vi "Median filter.vi"(11 "Rawdata":i32) -> (3 "Filtered element":i32)   [LabVIEW 2016]
doc: "Input\nRawdata\n\nOutput\nFiltered value\n\nThis VI implements a point to point median filter of rank 7. If one would like to change to the rank, you will need to set an odd number and change the size of the initial array for the feedback loop."
panel:
  in  "Middle":i32=4
  in  "Size of filter":i32=7
  # "Number of points to find median from,\nyou are best of choosing and odd number\nsince you want to avoid division on FPGA."
  # "Middle of size of filter"
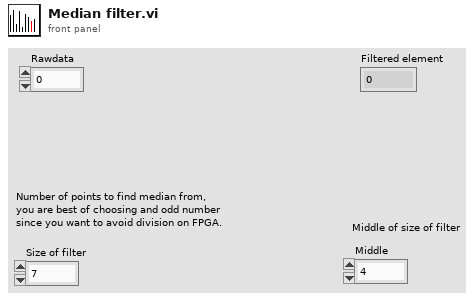
[diagram p1: front panel]
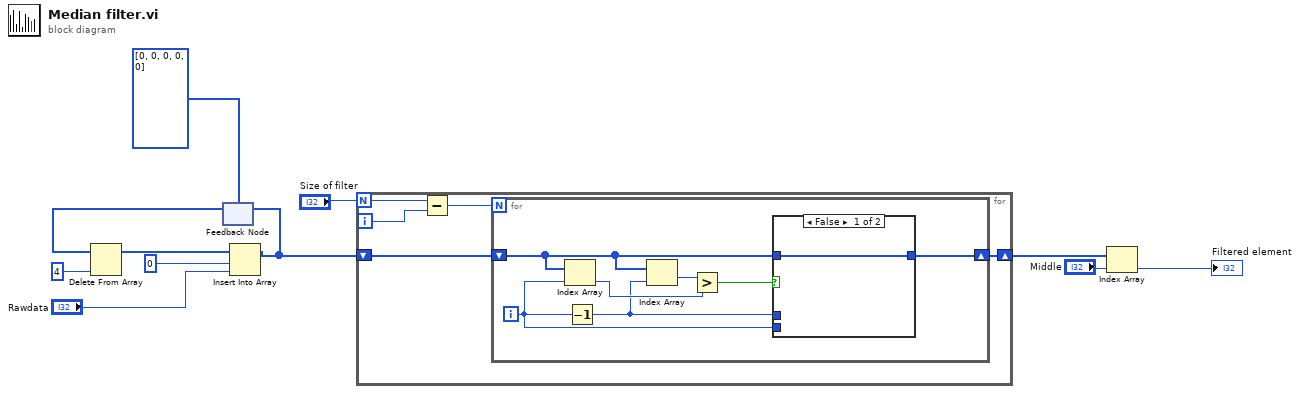
[diagram p0: block diagram]
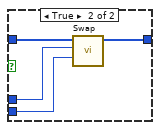
[diagram p2: hidden frame]
diagram:
  n1 = feedback #1(i32[] [0, 0, 0, 0, 0]) -> (w3:i32[])
  n2 = Delete From Array(array=w3, index=4) -> (array with subset deleted=w2:i32[])  [unwired: 1 in, 1 out]
  n3 = Insert Into Array(array=w2, index=0, new element="Rawdata") -> (w1:i32[])
  n4 = feedback-in #1(w1) -> ()
  n5 = for {
    N: "Size of filter" -> [w16]
    shift-right: [w12] -> w11
    shift-left: w1 -> [w13]
    i -> [w15]
    n6 = Subtract(x=w16, y=w15) -> (x-y=w14:i32)
    n7 = for {
      N: w14 -> [_]
      shift-right: [w19] -> w12
      shift-left: w13 -> [w23]
      i -> [w18]
      n8 = Index Array(array=w23, index=w18) -> (element=w21:i32)
      n9 = Decrement(x=w18) -> (x-1=w17:i32)
      n10 = Index Array(array=w23, index=w17) -> (element=w22:i32)
      n11 = Greater?(x=w22, y=w21) -> (0:w20:bool)
      n12 = case shown="False" w20 {
        tunnel: w23 -> [w24 w28]
        tunnel: w17 -> [_ w27]
        tunnel: w18 -> [_ w25]
        tunnel: [w24 w26] -> w19
        frame False {
        }
        frame True {
          n13 = call "Swap.vi"("Y"=w25, "X"=w27, "Unswapped Array"=w28) -> ("Swapped Array"=w26:i32[])  [unwired: 8 in]
        }
      }
    }
  }
  n14 = Index Array(array=w11, index="Middle") -> (element=→"Filtered element":i32)
